vi "Express VI - Append Signals.vi"() -> ()   [LabVIEW 2023]
doc: "Append Signals will append signals end to end in one of three ways, depending on what is wired to the Input Signals. \n\n1. If you have only wired Input Signal A, it will append all of the individual signals in A to each other, end to end, making one signal.\n2. If you have an individual signal on Input Signal B, it will be appended to the end of each signal in Input Signal A.\n3. If you have multiple signals on each input, it will append the first signal of B to the end of the first signal of A, the second signal of B to end of the second signal of A, etc.\n\nNote: \"Append only if t0 aligns and dt matches\" has been deselected on all three Append Signals Express VIs in this example. When selected, this option requires that the start of the appended signal (Input Signal B) must align with the end of the original signal (Input Signal A) and that they must have the same time between points (dt). When deselected, it no longer checks to ensure that either is true."
panel:
  out "Signal 1":dynamicdata(graph)
  in  "Tab Control":T1(tab)
  out "Append Signals Case 1":dynamicdata(graph)
  out "Signal 2":dynamicdata(graph)
  out "Append Signals Case 2":dynamicdata(graph)
  out "Signal 3":dynamicdata(graph)
  out "Append Signals Case 3":dynamicdata(graph)
  # "Overview: Demonstrates the use of the Append Signals Express VI.\nInstructions:\n1. Run the VI.\n2. Select each of the tabs in the tab control to learn about different ways to use the Append Signals Express VI."
  # "This is a combined signal. It is wired to Input Signal A in all three cases."
  # "In this case, the Append Signals Express VI has nothing wired to Input Signal B.  Input Signal A is a combined signal and the results are the two signals appended to each other."
  # "In this case, the Append Signals Express VI has a signal wired to Input Signal B.  Input Signal A is a combined signal and the result is a combined signal with the Input Signal B appended to each signal in Input Signal A."
  # "In this case, the Append Signals Express VI has combined signals wired to both of its inputs.  The result is a combined signal appended to another combined signal."
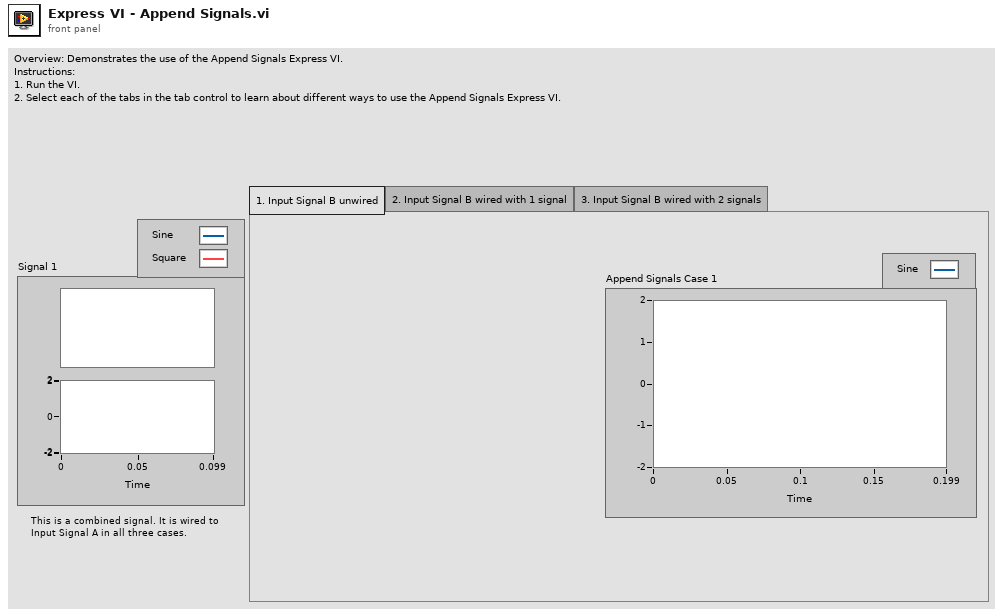
[diagram p1: front panel]
types:
  T1 = enum32{"1. Input Signal B unwired", "2. Input Signal B wired with 1 signal", "3. Input Signal B wired with 2 signals"}
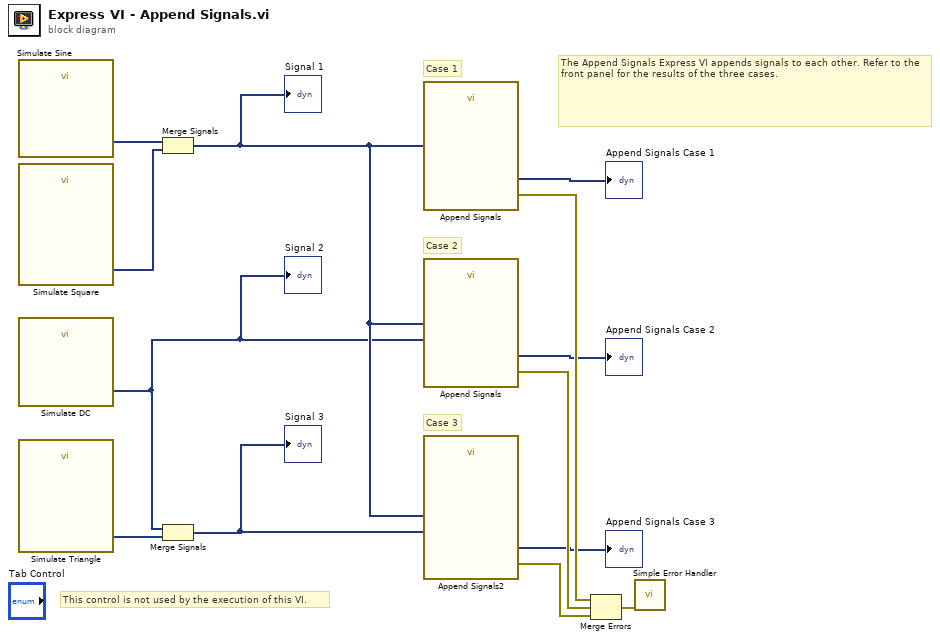
[diagram p0: block diagram]
diagram:
  # "The Append Signals Express VI appends signals to each other. Refer to the front panel for the results of the three cases."
  # "Case 3"
  # "Case 2"
  # "Case 1"
  # "This control is not used by the execution of this VI."
  n1 = call "Simulate Sine"() -> ("Sine"=w11:dynamicdata)  [unwired: 14 in, 1 out]
  n2 = call "Simulate Square"() -> ("Square"=w10:dynamicdata)  [unwired: 14 in, 1 out]
  n3 = call "Simulate DC"() -> ("DC with Uniform Noise"=w1:dynamicdata)  [unwired: 14 in, 1 out]
  "Signal 2" <- w1
  n4 = call "Simulate Triangle"() -> ("Triangle"=w9:dynamicdata)  [unwired: 14 in, 1 out]
  n5 = Merge Signals(w11, w10) -> (w6:dynamicdata)
  "Signal 1" <- w6
  n6 = Merge Signals(w1, w9) -> (w5:dynamicdata)
  "Signal 3" <- w5
  n7 = call "Append Signals"("Input Signal A"=w6) -> ("error out"=w12:errorcluster, "Appended Signals"=→"Append Signals Case 1":dynamicdata)  [unwired: 9 in]
  n8 = call "Append Signals"("Input Signal B"=w1, "Input Signal A"=w6) -> ("error out"=w13:errorcluster, "Appended Signals"=→"Append Signals Case 2":dynamicdata)  [unwired: 8 in]
  n9 = call "Append Signals2"("Input Signal B"=w5, "Input Signal A"=w6) -> ("error out"=w3:errorcluster, "Appended Signals"=→"Append Signals Case 3":dynamicdata)  [unwired: 8 in]
  n10 = Merge Errors(w12, w13, w3) -> (w2:errorcluster)
  n11 = call <vilib>:"Simple Error Handler.vi"("error in (no error)"=w2) -> ()  [unwired: 4 in, 5 out]
